vi "locker-Destroy.vi"(8 "error in (no error)":errorcluster, 11 "locker":refnum<queue>) -> (0 "error out":errorcluster)   [LabVIEW 2017]
doc: "Releases a locker created by locker-Create.vi. Call it once for every locker-Create."
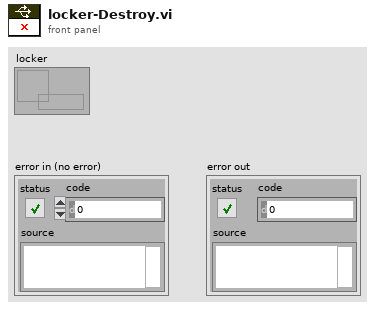
[diagram p1: front panel]
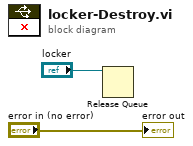
[diagram p0: block diagram]
diagram:
  n1 = Release Queue(queue="locker") -> ()  [unwired: 2 in, 3 out]
  "error out" <- "error in (no error)"
